vi "Find Project Folder.vi"(8 "error in (no error)":errorcluster, 11 "gScript Interpreter in":refnum<class "gScript Interpreter.lvclass">) -> (0 "error out":errorcluster, 3 "gScript Interpreter out":refnum<class "gScript Interpreter.lvclass">)   [LabVIEW 2017, in "gScript Interpreter.lvclass"]
uses:
  gScript Interpreter.lvclass
  gScript Interpreter.lvclass/gScript Interpreter.ctl
  <vilib>/Utility/config.llb/Read Key (Path).vi
  <vilib>/Utility/config.llb/Write Key (Path).vi
  <vilib>/Utility/config.llb/NI_LVConfig.lvlib
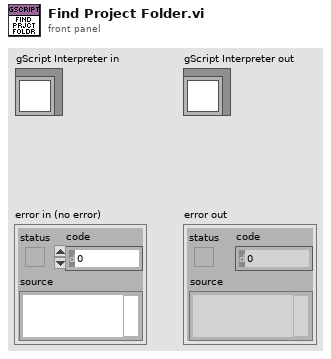
[diagram p1: front panel]
types:
  T1 = typedef "NI_LVConfig.lvlib/Config Data RefNum.ctl" = refnum<k1>
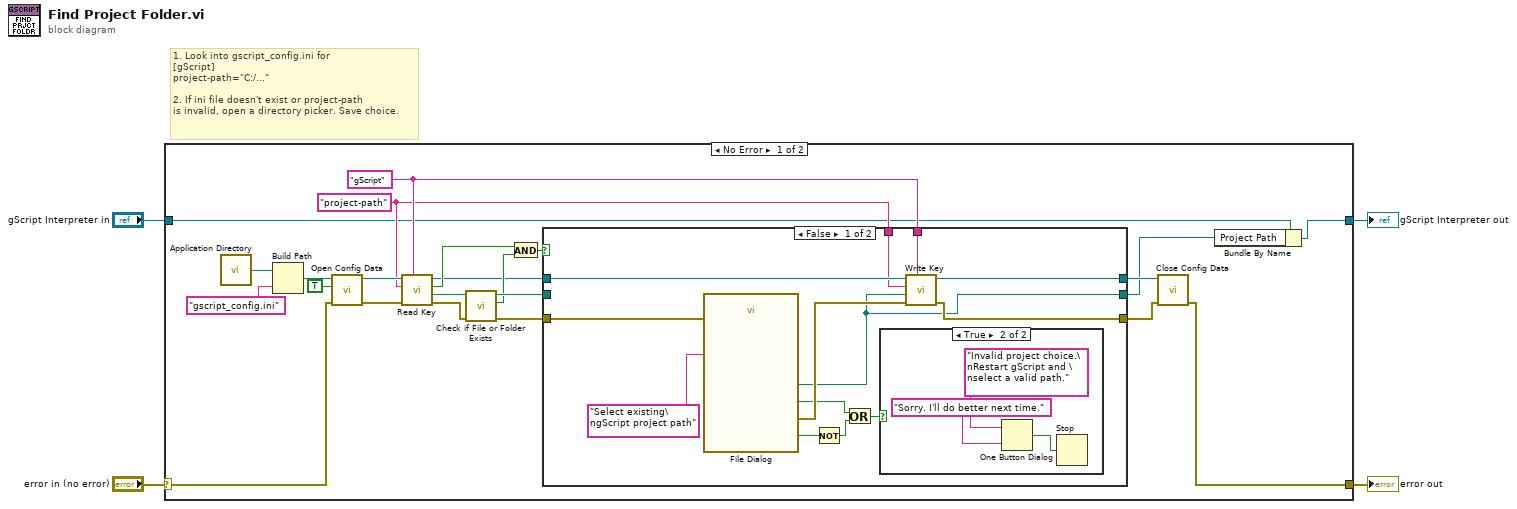
[diagram p0: block diagram]
diagram:
  # "1. Look into gscript_config.ini for \n[gScript]\nproject-path=\"C:/...\"\n\n2. If ini file doesn't exist or project-path\nis invalid, open a directory picker. Save choice."
  n1 = case shown="No Error" "error in (no error)" {
    selector: "error in (no error)" -> [w23 w48]
    tunnel: [w8 w48] -> w3
    tunnel: [w5 w47] -> w1
    tunnel: "gScript Interpreter in" -> [w7 w47]
    frame No Error {
      w11 = "project-path" ("key")
      w12 = "gScript" ("section")
      n2 = call <vilib>:"Application Directory.vi"() -> ("Application Directory"=w27:path)
      n3 = Build Path(base path=w27, name or relative path="gscript_config.ini") -> (appended path=w25:path)
      n4 = call <vilib>:"Open Config Data.vi"("error in (no error)"=w23, "create file if necessary (T)"=TRUE, "configuration file path"=w25) -> ("error out"=w22:errorcluster, "refnum"=w21:T1)  [unwired: 6 in, 1 out]
      n5 = call-poly <vilib>:"Read Key.vi"("section"=w12, "error in (no error)"=w22, "key"=w11, "refnum"=w21) -> ("error out"=w18:errorcluster, "value"=w20:path, "found?"=w17:bool, "refnum out"=w14:T1)  [unwired: 4 in]
      n6 = call <vilib>:"Check if File or Folder Exists.vi"("error in (no error)"=w18, "path"=w20) -> ("error out"=w13:errorcluster, "file or folder exists?"=w15:bool, "dup path"=w19:path)  [unwired: 7 in]
      n7 = And(x=w17, y=w15) -> (x .and. y?=w16:bool)
      n8 = case shown="False" w16 {
        tunnel: w19 -> [_ w46]
        tunnel: w14 -> [w37 w45]
        tunnel: [w32 w46] -> w6
        tunnel: w13 -> [w39 w44]
        tunnel: [w36 w45] -> w10
        tunnel: [w33 w44] -> w9
        tunnel: w12 -> [w35 _]
        tunnel: w11 -> [w34 _]
        frame False {
          n9 = call "File Dialog"("prompt"="Select existing\ngScript project path", "error in"=w39) -> ("selected path"=w32:path, "exists"=w31:bool, "cancelled"=w29:bool, "error out"=w38:errorcluster)  [unwired: 10 in]
          n10 = Not(x=w31) -> (.not. x?=w30:bool)
          n11 = Or(x=w29, y=w30) -> (x .or. y?=w28:bool)
          n12 = case shown="True" w28 {
            frame False {
            }
            frame True {
              n13 = One Button Dialog(message="Invalid project choice.\nRestart gScript and \nselect a valid path.", button name ("OK")="Sorry. I'll do better next time.") -> (true=w43:bool)
              n14 = Stop(stop? (T)=w43) -> ()
            }
          }
          n15 = call-poly <vilib>:"Write Key.vi"("section"=w35, "error in (no error)"=w38, "value"=w32, "key"=w34, "refnum"=w37) -> ("error out"=w33:errorcluster, "refnum out"=w36:T1)  [unwired: 4 in, 1 out]
        }
        frame True {
        }
      }
      n16 = call <vilib>:"Close Config Data.vi"("error in (no error)"=w9, "refnum"=w10) -> ("error out"=w8:errorcluster)  [unwired: 8 in, 1 out]
      n17 = Bundle By Name(cluster=w7, "Project Path"=w6) -> (w5:refnum<class "gScript Interpreter.lvclass">)
    }
    frame Error {
    }
  }
  "error out" <- w3
  "gScript Interpreter out" <- w1
